vi "蓄电池组通讯程序.vi"() -> ()   [LabVIEW 2010]
uses:
  <vilib>/Utility/NIReport.llb/NI_report.lvclass
  <vilib>/addons/_office/NI_ReportGenerationToolkit.lvlib
  <vilib>/Utility/NIReport.llb/Excel/NI_Excel.lvclass
  <vilib>/Instr/_visa.llb/VISA Configure Serial Port (Instr).vi
panel:
  out "字节数":u32
  out "充放电":string
  in  "文档保存":path
  out "开始放电":string
  in  "打开模板":path
  in  "打印份数":dbl
  in  "是否打印":bool
  out "放电起始":string
  out "串口设置":string
  out "当前计时":string
  in  "生成报表":bool
  in  "串口选择":refnum<visa-resource-name>
  in  "虚拟串口设置":bool
  in  "网传模块设置":bool
  in  "停止运行":bool
  out "通信异常":bool
  out "电池组别：":string
  out "布尔 2":bool
  out "电池组状态":string
  out "状态":string
  out "第24节":string
  out "第23节":string
  out "第22节":string
  out "第21节":string
  out "第20节":string
  out "第19节":string
  out "第18节":string
  out "第17节":string
  out "第16节":string
  out "第15节":string
  out "第14节":string
  out "第13节":string
  out "第12节":string
  out "第11节":string
  out "第10节":string
  out "第9节":string
  out "第8节":string
  out "第7节":string
  out "第6节":string
  out "第5节":string
  out "第4节":string
  out "第3节":string
  out "第2节":string
  out "第1节":string
  out "电压":string
  out "电流":string
  out "温度":string
  out "放电容量":string
  out "放电计时":string
  # "48V蓄电池组在线监测程序"
  # "适用于单体电池电压2V的24节蓄电池组"
  # "通讯设置"
  # "工作状态"
  # "V"
  # "Ah"
  # "A"
  # "℃"
  # "电池组工作状态"
  # "报表生成及打印"
  # "V"
  # "V"
  # "V"
  # "V"
  # "V"
  # "V"
  # "V"
  # "V"
  # "V"
  # "V"
  # "V"
  # "V"
  # "使用说明"
  # "V"
  # "V"
  # "V"
  # "V"
  # "1、启动检测程序后打开虚拟串口设置和网传模块设置程序，然后选择相应串口，一个串口对应一个电池组别。"
  # "2、如需打印或保存报表，应首先选择充、放电的标准模板，\n然后选择保存文件路径和设置文件名，选择是否打印和打印份数，点击生成报表，即可自动生成excel文档报表。"
  # "V"
  # "V"
  # "V"
  # "V"
  # "3、当系统工作于放电状态时，一旦蓄电池组或单体电池端\n电压达到设定临界点即发出声光告警，通过显示界面可查看\n相关数据。"
  # "V"
  # "V"
  # "V"
  # "V"
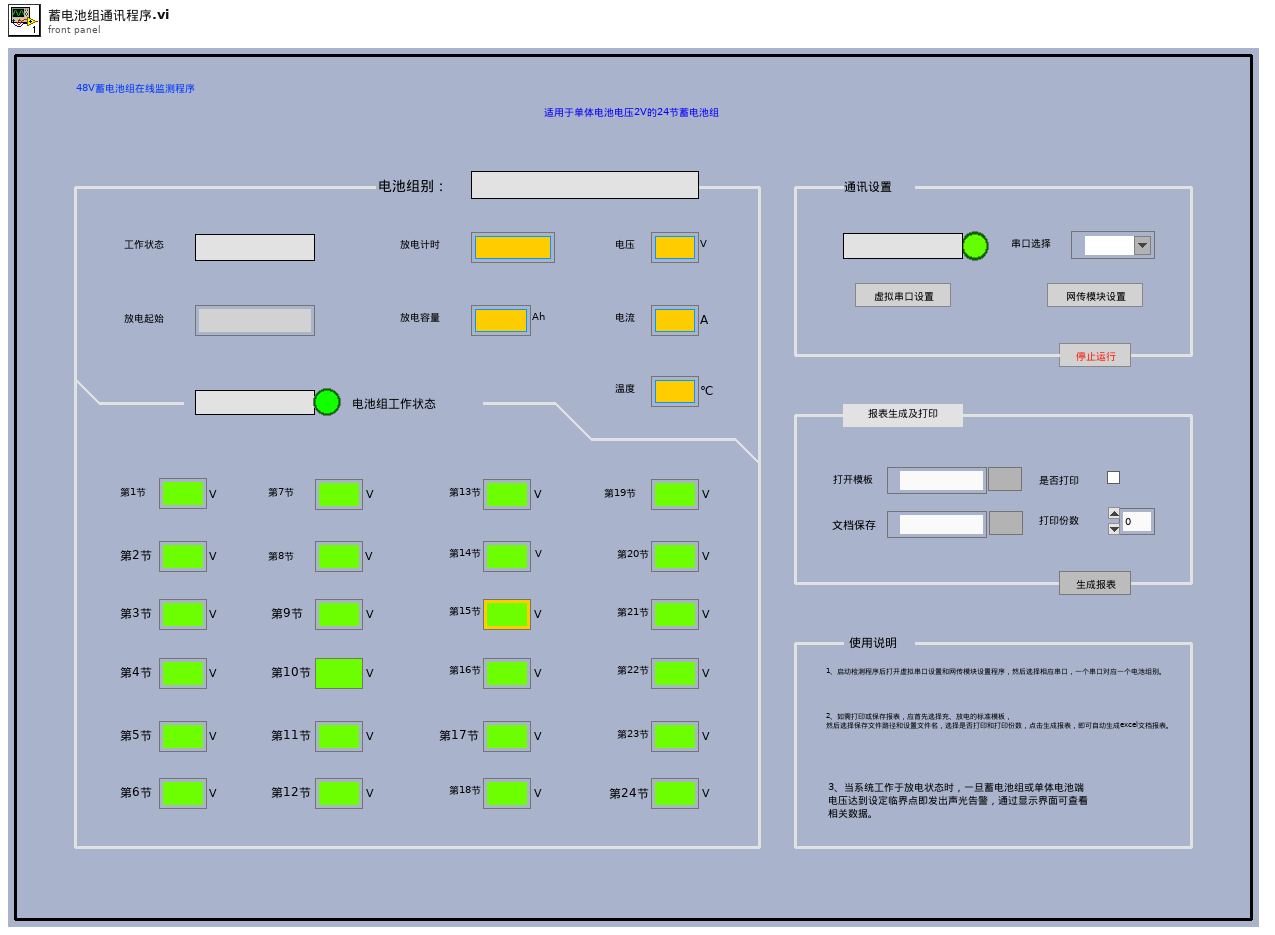
[diagram p1: front panel]
types:
  T1 = enum16{"Standard Report", "HTML", "Word", "Excel"}
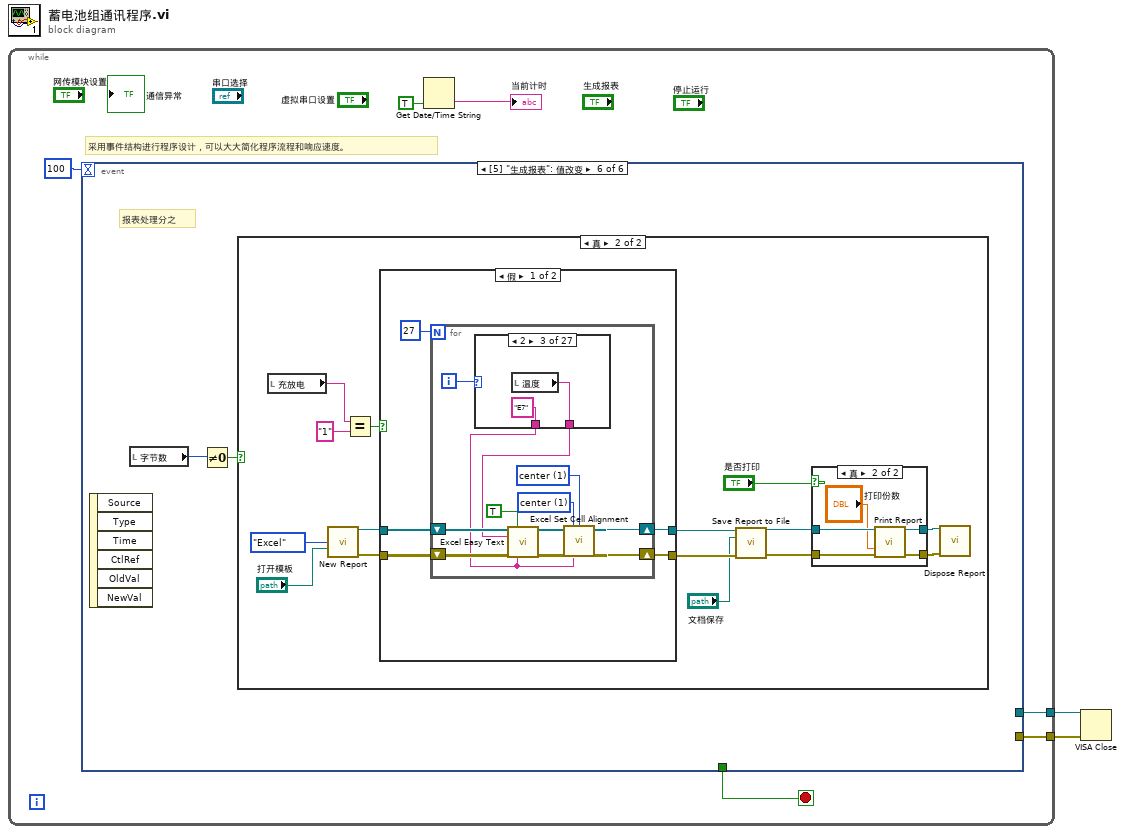
[diagram p0: block diagram]
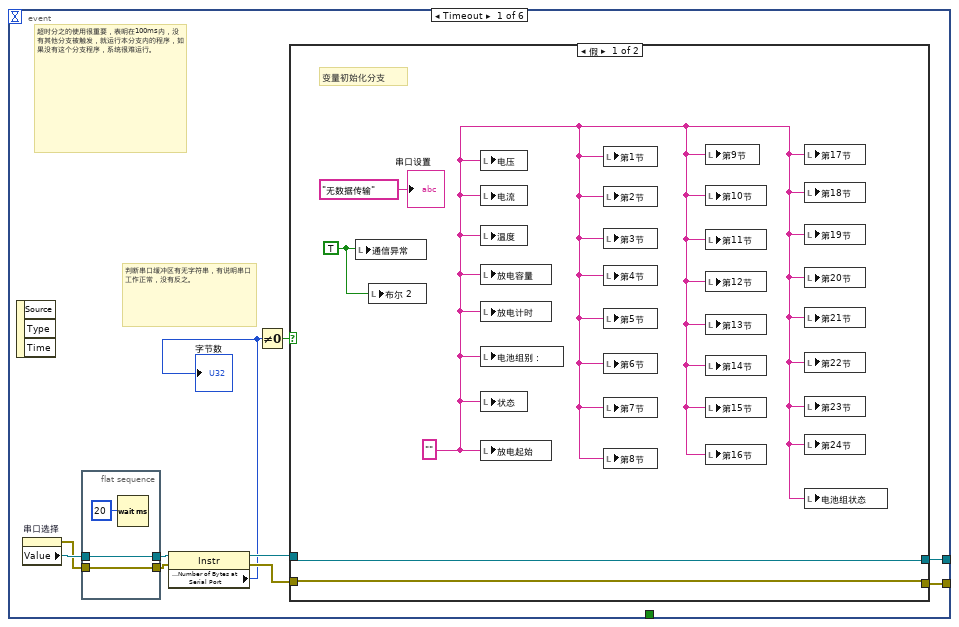
[diagram p2: hidden frame]
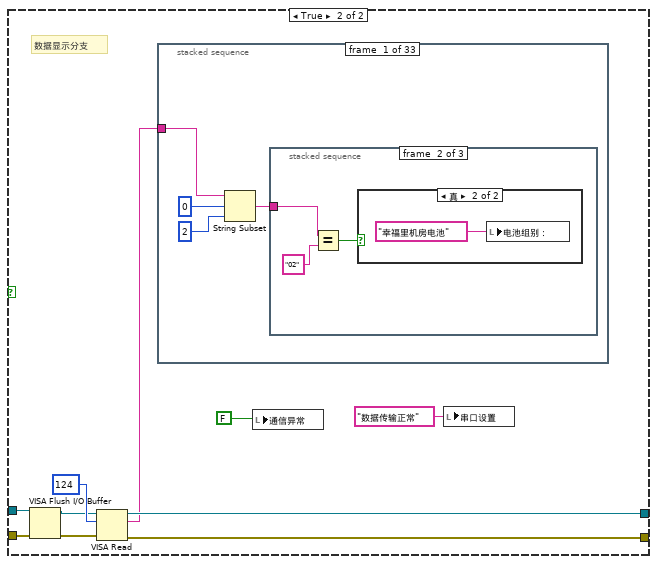
[diagram p3: hidden frame]
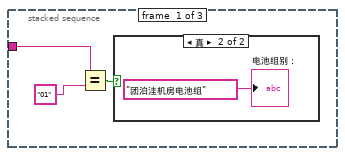
[diagram p4: hidden frame]
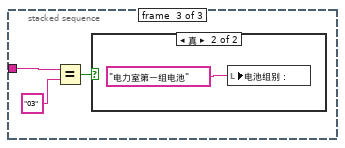
[diagram p7: hidden frame]
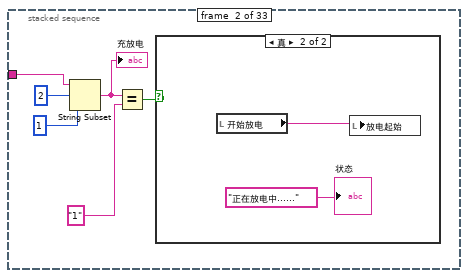
[diagram p9: hidden frame]
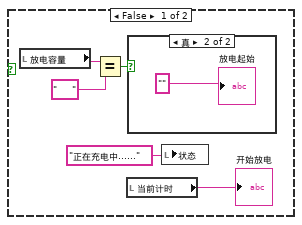
[diagram p10: hidden frame]
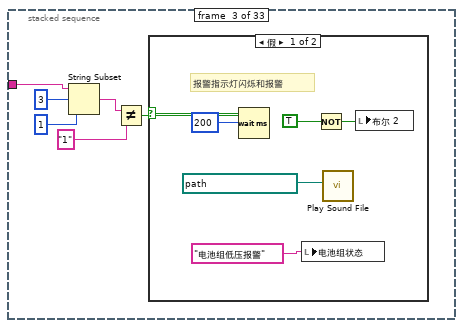
[diagram p12: hidden frame]
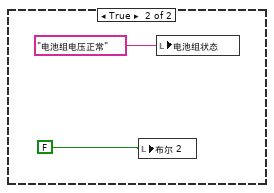
[diagram p13: hidden frame]
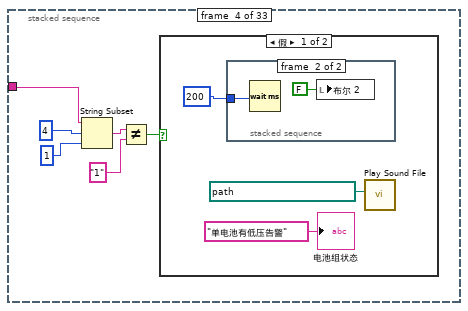
[diagram p14: hidden frame]
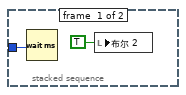
[diagram p15: hidden frame]
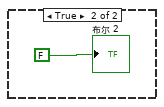
[diagram p16: hidden frame]
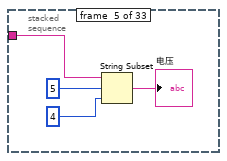
[diagram p17: hidden frame]
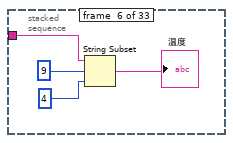
[diagram p18: hidden frame]
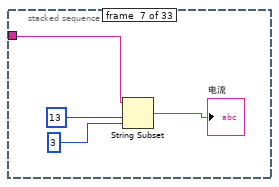
[diagram p19: hidden frame]
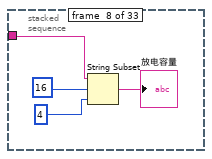
[diagram p20: hidden frame]
diagram:
  n1 = while {
    tunnel: [w4] -> w2
    tunnel: [w3] -> w1
    stop <- w8 stop-if-true
    # "采用事件结构进行程序设计，可以大大简化程序流程和响应速度。"
    n2 = event shown="[5] \"生成报表\": 值改变" {
      selector: _ -> [_ _ _ _ _ _]
      dyn-events: _ -> [_ _ _ _ _ _]
      timeout: 100 -> [_ _ _ _ _ _]
      tunnel: [_ w213 _ _ _ _] -> w8
      tunnel: [w15 _ _ _ _ _] -> w4
      tunnel: [w14 _ _ _ _ _] -> w3
      event Timeout {
        # "判断串口缓冲区有无字符串，有说明串口工作正常，没有反之。"
        # "超时分之的使用很重要，表明在100ms内，没有其他分支被触发，就运行本分支内的程序，如果没有这个分支程序，系统很难运行。"
        n3 = event-data() -> ()  [unwired: 1 in, 3 out]
        n4 = property on="串口选择" class="VISAName"() -> (error out=w10:errorcluster, "Value"=w12:refnum<visa-resource-name>)  [unwired: 2 in, 1 out]
        n5 = flat-sequence {
          tunnel: [w21] -> w13
          tunnel: w12 -> [w21]
          tunnel: w10 -> [w20]
          tunnel: [w20] -> w11
          frame #0 {
            n6 = Wait (ms)(milliseconds to wait=u32 20 ("等待时间（毫秒）")) -> ()  [unwired: 1 out]
          }
        }
        n7 = property class="Instr"(reference=w13, error in=w11) -> (reference out=w17:refnum<visa-resource-name>, error out=w16:errorcluster, "Serial Settings:Number of Bytes at Serial Port"=w9:u32)
        "字节数" <- w9
        n8 = Not Equal To 0?(x=w9) -> (x != 0?=w18:bool)
        n9 = case shown="假" w18 {
          tunnel: [w26 w33] -> w15
          tunnel: [w25 w32] -> w14
          tunnel: w17 -> [w26 w31]
          tunnel: w16 -> [w25 w30]
          frame False {
            w23 = TRUE ("值")
            w22 = ""
            # "变量初始化分支"
            n10 = local write "通信异常"(w23) -> ()
            n11 = local write "布尔 2"(w23) -> ()
            n12 = local write "电压"(w22) -> ()
            n13 = local write "电流"(w22) -> ()
            n14 = local write "温度"(w22) -> ()
            n15 = local write "放电容量"(w22) -> ()
            n16 = local write "放电计时"(w22) -> ()
            n17 = local write "电池组别："(w22) -> ()
            n18 = local write "状态"(w22) -> ()
            n19 = local write "放电起始"(w22) -> ()
            n20 = local write "第1节"(w22) -> ()
            n21 = local write "第2节"(w22) -> ()
            n22 = local write "第3节"(w22) -> ()
            n23 = local write "第4节"(w22) -> ()
            n24 = local write "第5节"(w22) -> ()
            n25 = local write "第6节"(w22) -> ()
            n26 = local write "第7节"(w22) -> ()
            n27 = local write "第8节"(w22) -> ()
            n28 = local write "第9节"(w22) -> ()
            n29 = local write "第10节"(w22) -> ()
            n30 = local write "第11节"(w22) -> ()
            n31 = local write "第12节"(w22) -> ()
            n32 = local write "第13节"(w22) -> ()
            n33 = local write "第14节"(w22) -> ()
            n34 = local write "第15节"(w22) -> ()
            n35 = local write "第16节"(w22) -> ()
            n36 = local write "第17节"(w22) -> ()
            n37 = local write "第18节"(w22) -> ()
            n38 = local write "第19节"(w22) -> ()
            n39 = local write "第20节"(w22) -> ()
            n40 = local write "第21节"(w22) -> ()
            n41 = local write "第22节"(w22) -> ()
            n42 = local write "第23节"(w22) -> ()
            n43 = local write "第24节"(w22) -> ()
            n44 = local write "电池组状态"(w22) -> ()
            "串口设置" <- "无数据传输" ("状态")
          }
          frame True {
            # "数据显示分支"
            n45 = VISA Flush I/O Buffer(VISA resource name=w31, error in (no error)=w30) -> (VISA resource name out=w35:refnum<visa-resource-name>, error out=w34:errorcluster)  [unwired: 1 in]
            n46 = VISA Read(VISA resource name=w35, byte count=u32 124 ("字节总数"), error in (no error)=w34) -> (VISA resource name out=w33:refnum<visa-resource-name>, read buffer=w29:string, error out=w32:errorcluster)  [unwired: 1 out]
            n47 = stacked-sequence {
              tunnel: w29 -> [w37 w53 w67 w81 w94 w99 w103 w106 w110 w114 w118 w122 w126 w130 w134 w138 w142 w146 w150 w154 w158 w162 w166 w170 w174 w178 w182 w186 w190 w194 w198 w202 w206]
              frame #0 {
                n48 = String Subset(string=w37, offset (0)=0 ("偏移量(0)"), length (rest)=2 ("长度（剩余）")) -> (substring=w38:string)
                n49 = stacked-sequence {
                  tunnel: w38 -> [w42 w47 w51]
                  frame #0 {
                    n50 = Equal?(x=w42, y="01") -> (x = y?=w43:bool)
                    n51 = case shown="真" w43 {
                      frame False {
                      }
                      frame True {
                        "电池组别：" <- "团泊洼机房电池组" ("电池回路")
                      }
                    }
                  }
                  frame #1 {
                    n52 = Equal?(x=w47, y="02") -> (x = y?=w45:bool)
                    n53 = case shown="真" w45 {
                      frame False {
                      }
                      frame True {
                        n54 = local write "电池组别："("幸福里机房电池" ("电池回路")) -> ()
                      }
                    }
                  }
                  frame #2 {
                    n55 = Equal?(x=w51, y="03") -> (x = y?=w49:bool)
                    n56 = case shown="真" w49 {
                      frame False {
                      }
                      frame True {
                        n57 = local write "电池组别："("电力室第一组电池" ("电池回路")) -> ()
                      }
                    }
                  }
                }
              }
              frame #1 {
                n58 = String Subset(string=w53, offset (0)=2 ("偏移量(0)"), length (rest)=1 ("长度（剩余）")) -> (substring=w58:string)
                "充放电" <- w58
                n59 = Equal?(x=w58, y="1") -> (x = y?=w54:bool)
                n60 = case shown="真" w54 {
                  frame False {
                    n61 = local read "放电容量"() -> (w60:string)
                    n62 = Equal?(x=w60, y="     ") -> (x = y?=w61:bool)
                    n63 = local read "当前计时"() -> (→"开始放电":string)
                    n64 = case shown="真" w61 {
                      frame False {
                      }
                      frame True {
                        "放电起始" <- "" ("放电起始")
                      }
                    }
                    n65 = local write "状态"("正在充电中......" ("当前工作状态")) -> ()
                  }
                  frame True {
                    n66 = local read "开始放电"() -> (w65:string)
                    n67 = local write "放电起始"(w65) -> ()
                    "状态" <- "正在放电中......" ("当前工作状态")
                  }
                }
              }
              frame #2 {
                n68 = String Subset(string=w67, offset (0)=3 ("偏移量(0)"), length (rest)=1 ("长度（剩余）")) -> (substring=w69:string)
                n69 = Not Equal?(x=w69, y="1") -> (x != y?=w68:bool)
                n70 = case shown="假" w68 {
                  frame False {
                    # "报警指示灯闪烁和报警"
                    n71 = Wait (ms)(milliseconds to wait=200) -> ()  [unwired: 1 out]
                    n72 = local write "电池组状态"("电池组低压报警" ("字符串")) -> ()
                    n73 = Not(x=TRUE ("布尔")) -> (.not. x?=w73:bool)
                    n74 = call <vilib>:"Play Sound File.vi"("path"=path "D:/National Instruments/LabVIEW 2014/我的文件/jingyin.wav") -> ()  [unwired: 9 in, 2 out]
                    n75 = local write "布尔 2"(w73) -> ()
                  }
                  frame True {
                    n76 = local write "布尔 2"(FALSE) -> ()
                    n77 = local write "电池组状态"("电池组电压正常" ("电池组低压警告")) -> ()
                  }
                }
              }
              frame #3 {
                n78 = String Subset(string=w81, offset (0)=4 ("偏移量(0)"), length (rest)=1 ("长度（剩余）")) -> (substring=w84:string)
                n79 = Not Equal?(x=w84, y="1") -> (x != y?=w82:bool)
                n80 = case shown="假" w82 {
                  frame False {
                    n81 = stacked-sequence {
                      tunnel: u32 200 ("等待时间（毫秒）") -> [w89 w91]
                      frame #0 {
                        n82 = Wait (ms)(milliseconds to wait=w89) -> ()  [unwired: 1 out]
                        n83 = local write "布尔 2"(TRUE ("布尔 2")) -> ()
                      }
                      frame #1 {
                        n84 = Wait (ms)(milliseconds to wait=w91) -> ()  [unwired: 1 out]
                        n85 = local write "布尔 2"(FALSE ("布尔 2")) -> ()
                      }
                    }
                    n86 = call <vilib>:"Play Sound File.vi"("path"=path "D:/National Instruments/LabVIEW 2014/我的文件/jingyin.wav") -> ()  [unwired: 9 in, 2 out]
                    "电池组状态" <- "单电池有低压告警" ("单电池低压告警")
                  }
                  frame True {
                    "布尔 2" <- FALSE ("布尔 2")
                  }
                }
              }
              frame #4 {
                n87 = String Subset(string=w94, offset (0)=5, length (rest)=4) -> (substring=→"电压":string)
              }
              frame #5 {
                n88 = String Subset(string=w99, offset (0)=9, length (rest)=4) -> (substring=→"温度":string)
              }
              frame #6 {
                n89 = String Subset(string=w103, offset (0)=13, length (rest)=3) -> (substring=→"电流":string)
              }
              frame #7 {
                n90 = String Subset(string=w106, offset (0)=16, length (rest)=4) -> (substring=→"放电容量":string)
              }
              frame #8 {
                n91 = String Subset(string=w110, offset (0)=20, length (rest)=8) -> (substring=→"放电计时":string)
              }
              frame #9 {
                n92 = String Subset(string=w114, offset (0)=28 ("偏移量(0)"), length (rest)=4 ("长度（剩余）")) -> (substring=→"第1节":string)
              }
              frame #10 {
                n93 = String Subset(string=w118, offset (0)=32 ("偏移量(0)"), length (rest)=4 ("长度（剩余）")) -> (substring=→"第2节":string)
              }
              frame #11 {
                n94 = String Subset(string=w122, offset (0)=36 ("偏移量(0)"), length (rest)=4 ("长度（剩余）")) -> (substring=→"第3节":string)
              }
              frame #12 {
                n95 = String Subset(string=w126, offset (0)=40 ("偏移量(0)"), length (rest)=4 ("长度（剩余）")) -> (substring=→"第4节":string)
              }
              frame #13 {
                n96 = String Subset(string=w130, offset (0)=44 ("偏移量(0)"), length (rest)=4 ("长度（剩余）")) -> (substring=→"第5节":string)
              }
              frame #14 {
                n97 = String Subset(string=w134, offset (0)=48 ("偏移量(0)"), length (rest)=4 ("长度（剩余）")) -> (substring=→"第6节":string)
              }
              frame #15 {
                n98 = String Subset(string=w138, offset (0)=52 ("偏移量(0)"), length (rest)=4 ("长度（剩余）")) -> (substring=→"第7节":string)
              }
              frame #16 {
                n99 = String Subset(string=w142, offset (0)=56 ("偏移量(0)"), length (rest)=4 ("长度（剩余）")) -> (substring=→"第8节":string)
              }
              frame #17 {
                n100 = String Subset(string=w146, offset (0)=60 ("偏移量(0)"), length (rest)=4 ("长度（剩余）")) -> (substring=→"第9节":string)
              }
              frame #18 {
                n101 = String Subset(string=w150, offset (0)=64 ("偏移量(0)"), length (rest)=4 ("长度（剩余）")) -> (substring=→"第10节":string)
              }
              frame #19 {
                n102 = String Subset(string=w154, offset (0)=68 ("偏移量(0)"), length (rest)=4 ("长度（剩余）")) -> (substring=→"第11节":string)
              }
              frame #20 {
                n103 = String Subset(string=w158, offset (0)=72 ("偏移量(0)"), length (rest)=4 ("长度（剩余）")) -> (substring=→"第12节":string)
              }
              frame #21 {
                n104 = String Subset(string=w162, offset (0)=76 ("偏移量(0)"), length (rest)=4 ("长度（剩余）")) -> (substring=→"第13节":string)
              }
              frame #22 {
                n105 = String Subset(string=w166, offset (0)=80 ("偏移量(0)"), length (rest)=4 ("长度（剩余）")) -> (substring=→"第14节":string)
              }
              frame #23 {
                n106 = String Subset(string=w170, offset (0)=84 ("偏移量(0)"), length (rest)=4 ("长度（剩余）")) -> (substring=→"第15节":string)
              }
              frame #24 {
                n107 = String Subset(string=w174, offset (0)=88 ("偏移量(0)"), length (rest)=4 ("长度（剩余）")) -> (substring=→"第16节":string)
              }
              frame #25 {
                n108 = String Subset(string=w178, offset (0)=92 ("偏移量(0)"), length (rest)=4 ("长度（剩余）")) -> (substring=→"第17节":string)
              }
              frame #26 {
                n109 = String Subset(string=w182, offset (0)=96 ("偏移量(0)"), length (rest)=4 ("长度（剩余）")) -> (substring=→"第18节":string)
              }
              frame #27 {
                n110 = String Subset(string=w186, offset (0)=100 ("偏移量(0)"), length (rest)=4 ("长度（剩余）")) -> (substring=→"第19节":string)
              }
              frame #28 {
                n111 = String Subset(string=w190, offset (0)=104 ("偏移量(0)"), length (rest)=4 ("长度（剩余）")) -> (substring=→"第20节":string)
              }
              frame #29 {
                n112 = String Subset(string=w194, offset (0)=108 ("偏移量(0)"), length (rest)=4 ("长度（剩余）")) -> (substring=→"第21节":string)
              }
              frame #30 {
                n113 = String Subset(string=w198, offset (0)=112 ("偏移量(0)"), length (rest)=4 ("长度（剩余）")) -> (substring=→"第22节":string)
              }
              frame #31 {
                n114 = String Subset(string=w202, offset (0)=116 ("偏移量(0)"), length (rest)=4 ("长度（剩余）")) -> (substring=→"第23节":string)
              }
              frame #32 {
                n115 = String Subset(string=w206, offset (0)=120 ("偏移量(0)"), length (rest)=4 ("长度（剩余）")) -> (substring=→"第24节":string)
              }
            }
            n116 = local write "通信异常"(FALSE ("值")) -> ()
            n117 = local write "串口设置"("数据传输正常" ("串口设置")) -> ()
          }
        }
      }
      event "停止运行": Value Change {
        w211 = TRUE ("通信异常")
        w212 = ""
        # "停止运行时再次进行变量初始化"
        n118 = event-data() -> ("NewVal"=w213:bool)  [unwired: 1 in, 5 out]
        n119 = local write "布尔 2"(w211) -> ()
        n120 = local write "通信异常"(w211) -> ()
        n121 = local write "电池组别："(w212) -> ()
        n122 = local write "放电容量"(w212) -> ()
        n123 = local write "放电计时"(w212) -> ()
        n124 = local write "温度"(w212) -> ()
        n125 = local write "电流"(w212) -> ()
        n126 = local write "电压"(w212) -> ()
        n127 = local write "放电起始"(w212) -> ()
        n128 = local write "状态"(w212) -> ()
        n129 = local write "电池组状态"(w212) -> ()
        n130 = local write "串口设置"("系统已停止运行" ("串口设置")) -> ()
        n131 = local write "第1节"(w212) -> ()
        n132 = local write "第2节"(w212) -> ()
        n133 = local write "第3节"(w212) -> ()
        n134 = local write "第4节"(w212) -> ()
        n135 = local write "第5节"(w212) -> ()
        n136 = local write "第6节"(w212) -> ()
        n137 = local write "第7节"(w212) -> ()
        n138 = local write "第8节"(w212) -> ()
        n139 = local write "第9节"(w212) -> ()
        n140 = local write "第10节"(w212) -> ()
        n141 = local write "第11节"(w212) -> ()
        n142 = local write "第12节"(w212) -> ()
        n143 = local write "第13节"(w212) -> ()
        n144 = local write "第14节"(w212) -> ()
        n145 = local write "第15节"(w212) -> ()
        n146 = local write "第16节"(w212) -> ()
        n147 = local write "第17节"(w212) -> ()
        n148 = local write "第18节"(w212) -> ()
        n149 = local write "第19节"(w212) -> ()
        n150 = local write "第20节"(w212) -> ()
        n151 = local write "第21节"(w212) -> ()
        n152 = local write "第22节"(w212) -> ()
        n153 = local write "第23节"(w212) -> ()
        n154 = local write "第24节"(w212) -> ()
      }
      event "虚拟串口设置": Value Change {
        n155 = event-data() -> ()  [unwired: 1 in, 6 out]
        n156 = call <vilib>:"System Exec.vi"("run minimized? (F)"=TRUE, "wait until completion? (T)"=FALSE, "command line"="D:\\VSP Management Software\\VSPMgr.exe") -> ()  [unwired: 5 in, 4 out]
      }
      event "网传模块设置": Value Change {
        n157 = event-data() -> ()  [unwired: 1 in, 6 out]
        n158 = call <vilib>:"System Exec.vi"("run minimized? (F)"=TRUE, "wait until completion? (T)"=FALSE, "command line"="D:\\VSP Management Software\\TCP.exe") -> ()  [unwired: 5 in, 4 out]
      }
      event "串口选择": Value Change {
        w220 = u16 10 items=["1.0"=10, "1.5"=15, "2.0"=20] ("stop bits (10: 1 bit)")
        # "使用事件结构处理串口初始化很好，可以保证只在改变串口时进行一次初始化，从而避免系统运行时端口的反复初始化。\n\n另外，尝试发现，串口初始化可以脱离数据管道运行，而超时里的语句则是运行的关键了！"
        n159 = event-data() -> ("NewVal"=w223:refnum<visa-resource-name>)  [unwired: 1 in, 5 out]
        n160 = call-poly "VISA Configure Serial Port"("VISA resource name"=w223, "timeout (10sec)"=u32 100, "baud rate (9600)"=38400, "data bits (8)"=u16 8, "parity (0:none)"=enum16{"None", "Odd", "Even", "Mark", "Space"}."None", "stop bits (10: 1 bit)"=w220) -> ()  [unwired: 8 in, 2 out]
      }
      event "生成报表": Value Change {
        # "报表处理分之"
        n161 = event-data() -> ()  [unwired: 1 in, 6 out]
        n162 = local read "字节数"() -> (w226:u32)
        n163 = Not Equal To 0?(x=w226) -> (x != 0?=w227:bool)
        n164 = case shown="真" w227 {
          frame False {
            n165 = call "显示对话框信息"("Message"="对不起，无数据传输时不能处理报表请求") -> ()  [unwired: 9 in, 2 out]
          }
          frame True {
            n166 = local read "充放电"() -> (w230:string)
            n167 = call <vilib>:"New Report.vi"("report type"=T1."Excel", "template (empty)"="打开模板") -> ("report out"=w237:refnum<class "NI_report.lvclass">, "error out"=w232:errorcluster)  [unwired: 12 in]
            n168 = Equal?(x=w230, y="1") -> (x = y?=w234:bool)
            n169 = case shown="假" w234 {
              tunnel: w237 -> [w245 w319]
              tunnel: w232 -> [w244 w318]
              tunnel: [w247 w317] -> w236
              tunnel: [w246 w316] -> w235
              frame False {
                n170 = for {
                  N: 27 -> [_]
                  shift-right: [w260] -> w247
                  shift-left: w245 -> [w256]
                  shift-right: [w259] -> w246
                  shift-left: w244 -> [w255]
                  i -> [w249]
                  w250 = 1 items=["left", "center", "right"] ("horizontal alignment (left)")
                  w251 = 1 items=["top", "center", "bottom"] ("vertical alignment (top)")
                  n171 = case shown="2" w249 {
                    tunnel: ["A7" "C7" "E7" "B9" "B10" "B11" "B12" "B13" "B14" "B15" "B16" "D9" "D10" "D11" "D12" "D13" "D14" "D15" "D16" "F9" "F10" "F11" "F12" "F13" "F14" "F15" "F16"] -> w254
                    tunnel: [w261 w263 w265 w268 w270 w272 w274 w276 w278 w280 w282 w284 w286 w288 w290 w292 w294 w296 w298 w299 w302 w303 w306 w308 w310 w312 w314] -> w253
                    frame 0, Default {
                      n172 = local read "电压"() -> (w261:string)
                    }
                    frame 1 {
                      n173 = local read "电流"() -> (w263:string)
                    }
                    frame 2 {
                      n174 = local read "温度"() -> (w265:string)
                    }
                    frame 3 {
                      n175 = local read "第1节"() -> (w268:string)
                    }
                    frame 4 {
                      n176 = local read "第2节"() -> (w270:string)
                    }
                    frame 5 {
                      n177 = local read "第3节"() -> (w272:string)
                    }
                    frame 6 {
                      n178 = local read "第4节"() -> (w274:string)
                    }
                    frame 7 {
                      n179 = local read "第5节"() -> (w276:string)
                    }
                    frame 8 {
                      n180 = local read "第6节"() -> (w278:string)
                    }
                    frame 9 {
                      n181 = local read "第7节"() -> (w280:string)
                    }
                    frame 10 {
                      n182 = local read "第8节"() -> (w282:string)
                    }
                    frame 11 {
                      n183 = local read "第9节"() -> (w284:string)
                    }
                    frame 12 {
                      n184 = local read "第10节"() -> (w286:string)
                    }
                    frame 13 {
                      n185 = local read "第11节"() -> (w288:string)
                    }
                    frame 14 {
                      n186 = local read "第12节"() -> (w290:string)
                    }
                    frame 15 {
                      n187 = local read "第13节"() -> (w292:string)
                    }
                    frame 16 {
                      n188 = local read "第14节"() -> (w294:string)
                    }
                    frame 17 {
                      n189 = local read "第15节"() -> (w296:string)
                    }
                    frame 18 {
                      n190 = local read "第16节"() -> (w298:string)
                    }
                    frame 19 {
                      n191 = local read "第17节"() -> (w299:string)
                    }
                    frame 20 {
                      n192 = local read "第18节"() -> (w302:string)
                    }
                    frame 21 {
                      n193 = local read "第19节"() -> (w303:string)
                    }
                    frame 22 {
                      n194 = local read "第20节"() -> (w306:string)
                    }
                    frame 23 {
                      n195 = local read "第21节"() -> (w308:string)
                    }
                    frame 24 {
                      n196 = local read "第22节"() -> (w310:string)
                    }
                    frame 25 {
                      n197 = local read "第23节"() -> (w312:string)
                    }
                    frame 26 {
                      n198 = local read "第24节"() -> (w314:string)
                    }
                  }
                  n199 = call <vilib>:"Excel Easy Text.vi"("report in"=w256, "border? (F)"=TRUE, "text"=w253, "error in (no error)"=w255, "name (\"\")"=w254) -> ("report out"=w258:refnum<class "NI_report.lvclass">, "error out"=w257:errorcluster)  [unwired: 6 in, 3 out]
                  n200 = call <vilib>:"Excel Set Cell Alignment.vi"("report in"=w258, "vertical alignment (top)"=w251, "horizontal alignment (left)"=w250, "error in (no error)"=w257, "name (\"\")"=w254) -> ("report out"=w260:refnum<class "NI_report.lvclass">, "error out"=w259:errorcluster)  [unwired: 9 in]
                }
              }
              frame True {
                n201 = for {
                  N: 30 -> [_]
                  shift-right: [w324] -> w317
                  shift-left: w319 -> [w326]
                  shift-right: [w323] -> w316
                  shift-left: w318 -> [w325]
                  i -> [w320]
                  w330 = 1 items=["top", "center", "bottom"] ("vertical alignment (top)")
                  w329 = 1 items=["left", "center", "right"] ("horizontal alignment (left)")
                  n202 = case shown="2" w320 {
                    tunnel: [w333 w334 w336 w338 w340 w342 w344 w346 w348 w351 w352 w354 w356 w358 w360 w363 w364 w367 w368 w370 w372 w374 w376 w378 w381 w383 w385 w387 w388 w390] -> w321
                    tunnel: ["A7" ("name (\"\")") "B7" "C7" ("name (\"\")") "D7" ("name (\"\")") "E7" ("name (\"\")") "F7" ("name (\"\")") "B9" ("name (\"\")") "B10" ("name (\"\")") "B11" ("name (\"\")") "B12" ("name (\"\")") "B13" ("name (\"\")") "B14" ("name (\"\")") "B15" ("name (\"\")") "B16" ("name (\"\")") "D9" ("name (\"\")") "D10" ("name (\"\")") "D11" ("name (\"\")") "D12" ("name (\"\")") "D13" ("name (\"\")") "D14" ("name (\"\")") "D15" ("name (\"\")") "D16" ("name (\"\")") "F9" ("name (\"\")") "F10" ("name (\"\")") "F11" ("name (\"\")") "F12" ("name (\"\")") "F13" ("name (\"\")") "F14" ("name (\"\")") "F15" ("name (\"\")") "F16" ("name (\"\")")] -> w322
                    frame 0, Default {
                      n203 = local read "电压"() -> (w333:string)
                    }
                    frame 1 {
                      n204 = local read "电流"() -> (w334:string)
                    }
                    frame 2 {
                      n205 = local read "温度"() -> (w336:string)
                    }
                    frame 3 {
                      n206 = local read "放电容量"() -> (w338:string)
                    }
                    frame 4 {
                      n207 = local read "放电计时"() -> (w340:string)
                    }
                    frame 5 {
                      n208 = local read "放电起始"() -> (w342:string)
                    }
                    frame 6 {
                      n209 = local read "第1节"() -> (w344:string)
                    }
                    frame 7 {
                      n210 = local read "第2节"() -> (w346:string)
                    }
                    frame 8 {
                      n211 = local read "第3节"() -> (w348:string)
                    }
                    frame 9 {
                      n212 = local read "第4节"() -> (w351:string)
                    }
                    frame 10 {
                      n213 = local read "第5节"() -> (w352:string)
                    }
                    frame 11 {
                      n214 = local read "第6节"() -> (w354:string)
                    }
                    frame 12 {
                      n215 = local read "第7节"() -> (w356:string)
                    }
                    frame 13 {
                      n216 = local read "第8节"() -> (w358:string)
                    }
                    frame 14 {
                      n217 = local read "第9节"() -> (w360:string)
                    }
                    frame 15 {
                      n218 = local read "第10节"() -> (w363:string)
                    }
                    frame 16 {
                      n219 = local read "第11节"() -> (w364:string)
                    }
                    frame 17 {
                      n220 = local read "第12节"() -> (w367:string)
                    }
                    frame 18 {
                      n221 = local read "第13节"() -> (w368:string)
                    }
                    frame 19 {
                      n222 = local read "第14节"() -> (w370:string)
                    }
                    frame 20 {
                      n223 = local read "第15节"() -> (w372:string)
                    }
                    frame 21 {
                      n224 = local read "第16节"() -> (w374:string)
                    }
                    frame 22 {
                      n225 = local read "第17节"() -> (w376:string)
                    }
                    frame 23 {
                      n226 = local read "第18节"() -> (w378:string)
                    }
                    frame 24 {
                      n227 = local read "第19节"() -> (w381:string)
                    }
                    frame 25 {
                      n228 = local read "第20节"() -> (w383:string)
                    }
                    frame 26 {
                      n229 = local read "第21节"() -> (w385:string)
                    }
                    frame 27 {
                      n230 = local read "第22节"() -> (w387:string)
                    }
                    frame 28 {
                      n231 = local read "第23节"() -> (w388:string)
                    }
                    frame 29 {
                      n232 = local read "第24节"() -> (w390:string)
                    }
                  }
                  n233 = call <vilib>:"Excel Easy Text.vi"("report in"=w326, "border? (F)"=TRUE, "text"=w321, "error in (no error)"=w325, "name (\"\")"=w322) -> ("report out"=w328:refnum<class "NI_report.lvclass">, "error out"=w327:errorcluster)  [unwired: 6 in, 3 out]
                  n234 = call <vilib>:"Excel Set Cell Alignment.vi"("report in"=w328, "vertical alignment (top)"=w330, "horizontal alignment (left)"=w329, "error in (no error)"=w327, "name (\"\")"=w322) -> ("report out"=w324:refnum<class "NI_report.lvclass">, "error out"=w323:errorcluster)  [unwired: 9 in]
                }
              }
            }
            n235 = call-dynamic "Save Report to File.vi"("report in"=w236, "report file path"="文档保存", "error in (no error)"=w235) -> ("report out"=w242:refnum<class "NI_report.lvclass">, "error out"=w241:errorcluster)  [unwired: 11 in]
            n236 = case shown="真" "是否打印" {
              tunnel: w242 -> [w393 w398]
              tunnel: w241 -> [w392 w397]
              tunnel: [w392 w396] -> w240
              tunnel: [w393 w395] -> w239
              frame False {
              }
              frame True {
                n237 = call-dynamic "Print Report.vi"("report in"=w398, "number of copies (1)"="打印份数", "error in (no error)"=w397) -> ("report out"=w395:refnum<class "NI_report.lvclass">, "error out"=w396:errorcluster)  [unwired: 11 in]
              }
            }
            n238 = call-dynamic "Dispose Report.vi"("report in"=w239, "error in (no error)"=w240) -> ()  [unwired: 13 in, 1 out]
          }
        }
      }
    }
    n239 = Get Date/Time String(want seconds? (F)=TRUE ("需要秒？(F)")) -> (time string=→"当前计时":string)  [unwired: 2 in, 1 out]
  }
  n240 = VISA Close(VISA resource name=w2, error in (no error)=w1) -> ()  [unwired: 1 out]
